vi "init.vi"(8 "error in (no error)":errorcluster, 11 "Protocol_Logging in":refnum<class "Protocol_Logging.lvclass">) -> (0 "error out":errorcluster, 3 "Protocol_Logging out":refnum<class "Protocol_Logging.lvclass">)   [LabVIEW 2011, in "Protocol_Logging.lvclass"]
uses:
  Protocol_Logging.lvclass
  protocol_Generic/Protocol_Generic.lvclass
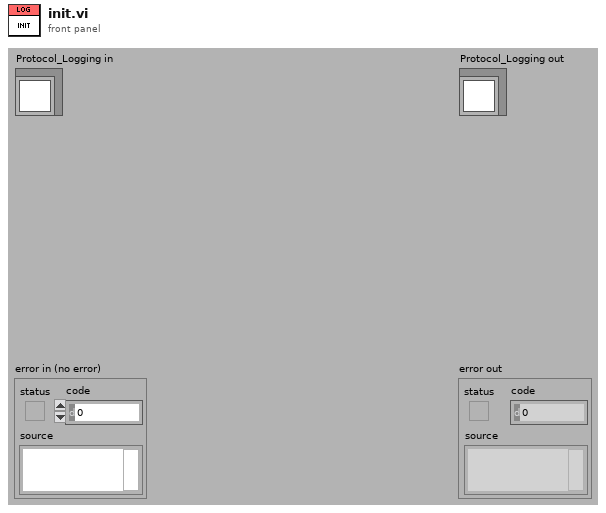
[diagram p1: front panel]
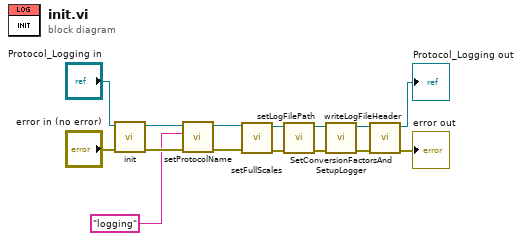
[diagram p0: block diagram]
diagram:
  n1 = call-parent "init.vi"("error in (no error)"="error in (no error)", "Protocol_Generic in"="Protocol_Logging in") -> ("error out"=w3:errorcluster, "Protocol_Generic out"=w4:refnum<class "Protocol_Logging.lvclass">)  [unwired: 8 in]
  n2 = call-dynamic "setProtocolName.vi"("error in (no error)"=w3, "Name"="logging", "Protocol_Generic in"=w4) -> ("error out"=w5:errorcluster, "Protocol_Generic out"=w2:refnum<class "Protocol_Logging.lvclass">)  [unwired: 7 in]
  n3 = call "setFullScales.vi"("error out 2"=w5, "Protocol_Generic out 2"=w2) -> ("error out"=w12:errorcluster, "Protocol_Generic out"=w13:refnum<class "Protocol_Logging.lvclass">)  [unwired: 8 in]
  n4 = call "setLogFilePath.vi"("error in (no error)"=w12, "Protocol_Generic out 2"=w13) -> ("error out"=w9:errorcluster, "Protocol_Generic out"=w7:refnum<class "Protocol_Logging.lvclass">)  [unwired: 8 in]
  n5 = call "SetConversionFactorsAndSetupLogger.vi"("error out 2"=w9, "Protocol_Generic out 2"=w7) -> ("error out"=w8:errorcluster, "Protocol_Generic out"=w6:refnum<class "Protocol_Logging.lvclass">)  [unwired: 8 in]
  n6 = call "writeLogFileHeader.vi"("error out 2"=w8, "Protocol_Generic out"=w6) -> ("error out"=→"error out":errorcluster, "Protocol_Generic out 2"=→"Protocol_Logging out":refnum<class "Protocol_Logging.lvclass">)  [unwired: 8 in]
